vi "Write Configuration Path.vi"(8 "error in (no error)":errorcluster, 10 "name or relative path":string, 11 "Instrument in":refnum<class "Instrument.lvclass">) -> (0 "error out":errorcluster, 3 "Instrument out":refnum<class "Instrument.lvclass">)   [LabVIEW 2016, in "Instrument.lvclass"]
uses:
  Instrument.lvclass
  <vilib>/Utility/sysdir.llb/System Directory Type.ctl
  Instrument.lvclass/Instrument.ctl
  Configuration/Configuration.lvclass
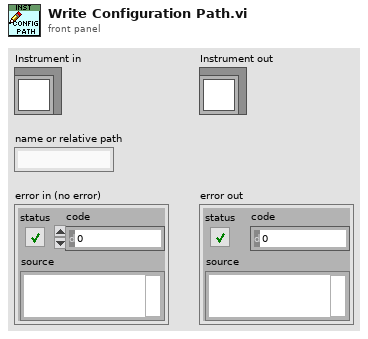
[diagram p1: front panel]
types:
  T1 = typedef "System Directory Type.ctl" = i32
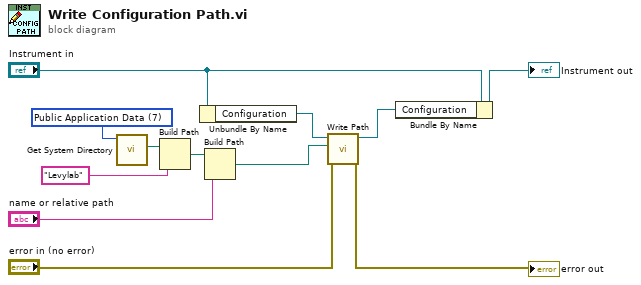
[diagram p0: block diagram]
diagram:
  w8 = T1 7 items=["User Home"=0, "User Desktop"=1, "User Documents"=2, "User Application Data"=3, "User Preferences"=4, "User Temporary"=5, "Public Documents"=6, "Public Application Data"=7, "Public Preferences"=8, "Public Cache"=13, "System Core Libraries"=9, "System Installed Libraries"=10, "Application Files"=11, "Boot Volume Root"=12] ("system directory type")
  n1 = call <vilib>:"Get System Directory.vi"("system directory type"=w8) -> ("system directory"=w5:path)  [unwired: 10 in]
  n2 = Build Path(base path=w5, name or relative path="Levylab") -> (appended path=w7:path)
  n3 = Unbundle By Name("Instrument in") -> ("Configuration"=w1:refnum<class "Configuration.lvclass">)
  n4 = Build Path(base path=w7, name or relative path="name or relative path") -> (appended path=w9:path)
  n5 = call-dynamic "Write Path.vi"("error in (no error)"="error in (no error)", "Path"=w9, "Configuration in"=w1) -> ("error out"=→"error out":errorcluster, "Configuration out"=w2:refnum<class "Configuration.lvclass">)  [unwired: 7 in]
  n6 = Bundle By Name(cluster="Instrument in", "Configuration"=w2) -> (→"Instrument out":refnum<class "Instrument.lvclass">)
